vi "Harmonics MSMT Configure Fetch Evaluations.vi"(8 "error in (no error)":errorcluster, 9 "SA Pin":string="SA PIN", 10 "Harmonic":i8, 11 "Harmonics in":refnum<class "Harmonics.lvclass">) -> (0 "error out":errorcluster, 1 "Exported Data Location":string, 2 "Array":T1[](array[typedef]) {"Low Limit" format="%#_13g"; "SI Scaling" items=["femto"=-15, "pico"=-12, "nano"=-9, "micro"=-6, "milli"=-3, "percent"=-2, ""=0, "kilo"=3, "mega"=6, "giga"=9, "tera"=12]}, 3 "Harmonics out":refnum<class "Harmonics.lvclass">)   [LabVIEW 2018, in "Harmonics.lvlib" / "Harmonics.lvclass"]
uses:
  Harmonics.lvclass
  C:/Sequence Automation/Plugins/Measurement Interface.lvlibp/Measurement Interface.lvclass
  Plugins/TestStand API Tools (TSAT).lvlibp/Evaluation Actions/Includes/Controls/TSAT Evaluation.ctl
  Plugins/TestStand API Tools (TSAT).lvlibp/Evaluation Actions/Includes/Controls/TSAT Eval SI Unit Scaling.ctl
  Plugins/TestStand API Tools (TSAT).lvlibp/Evaluation Actions/Includes/Controls/TSAT Evaluation Type.ctl
  Plugins/SeqAuto IEvaluation.lvlibp/SeqAuto IEvaluation.lvclass
  Harmonics.lvclass/Harmonics.ctl
  Evaluations/Harmonics/Harmonics_CHP/Harmonics_CHP.lvclass/Harmonics_CHP.ctl
  Protected Methods/Read DC Pins.vi
  Evaluations/Harmonics/Harmonics_CHP/Read Exported Data Location.vi
  Evaluations/DC Evaluations/DC_IDD.lvclass
  C:/Sequence Automation/Plugins/SeqAuto IEvaluation.lvlibp/SeqAuto IEvaluation.lvclass
  Plugins/Measurement Interface.lvlibp/Private Methods/Measurement Name/Read Measurement Name.vi
  Plugins/Measurement Interface.lvlibp/Private Methods/Measurement Parameters/Read Measurement Parameters.vi
  Plugins/String Database.lvlibp/String Database.lvclass
  Evaluations/Harmonics/Harmonics_CHP/Harmonics_CHP.lvclass
  Plugins/TestStand API Tools (TSAT).lvlibp/Evaluation Actions/TSAT Evaluation Actions.lvlib
  Plugins/Test Number and Bin Generator.lvlibp/Test Number and Bin Generator/Test Number and Bin Generator.lvclass
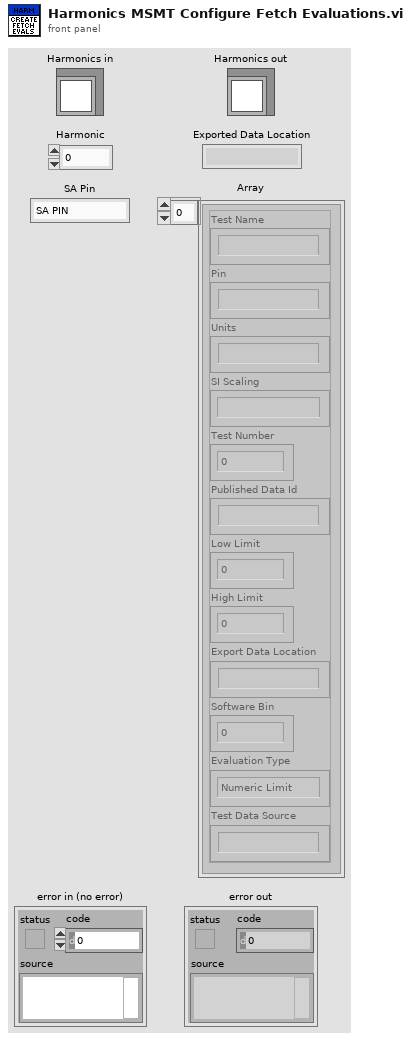
[diagram p1: front panel]
types:
  T1 = typedef "TestStand API Tools (TSAT).lvlibp/TSAT Evaluation Actions.lvlib/TSAT Evaluation.ctl" = cluster{"Test Name":string, "Pin":string, "Units":string, "SI Scaling":T2, "Test Number":i32, "Published Data Id":string, "Low Limit":dbl, "High Limit":dbl, "Export Data Location":string, "Software Bin":i64, "Evaluation Type":T3, "Test Data Source":string}
  T2 = typedef "TestStand API Tools (TSAT).lvlibp/TSAT Evaluation Actions.lvlib/TSAT Eval SI Unit Scaling.ctl" = i16
  T3 = typedef "TestStand API Tools (TSAT).lvlibp/TSAT Evaluation Actions.lvlib/TSAT Evaluation Type.ctl" = enum16{"Numeric Limit", "Pass/Fail", "None"}
  T4 = typedef "Test Number and Bin Generator.lvlibp/Test Number and Bin Generator.lvclass/Session Handle.ctl" = refnum<data-value>
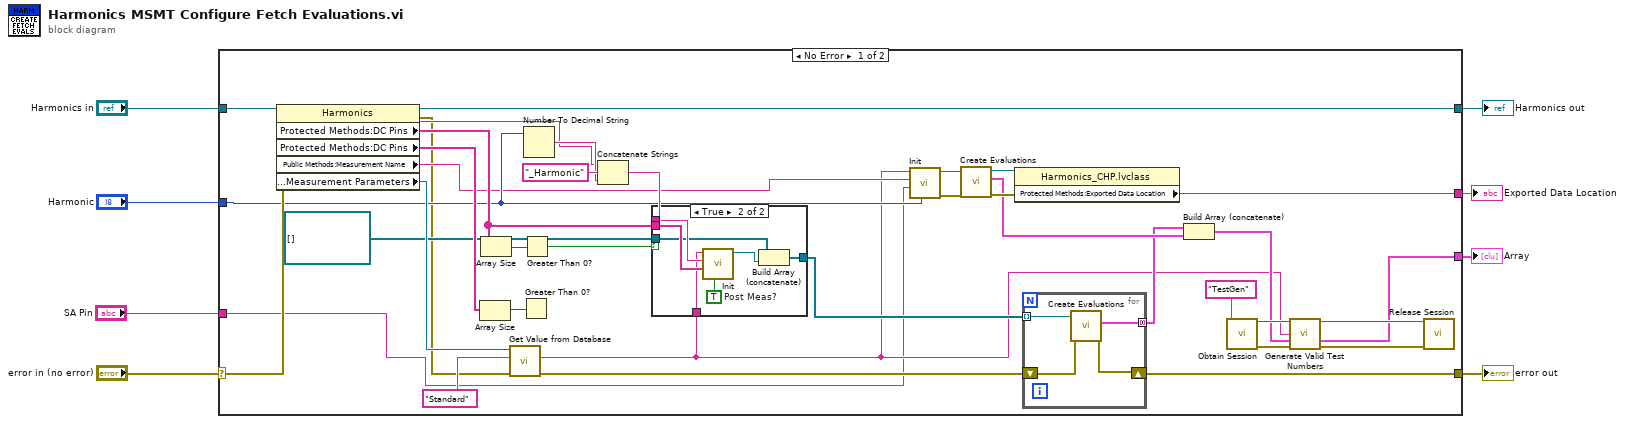
[diagram p0: block diagram]
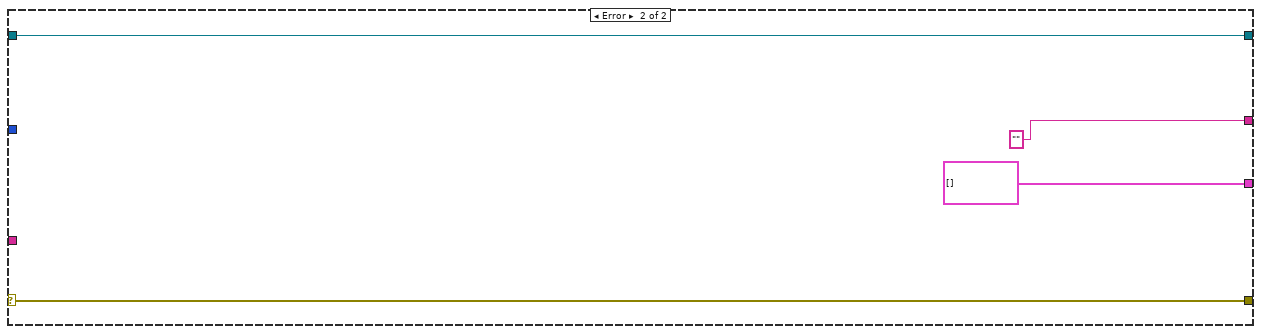
[diagram p3: hidden frame]
diagram:
  n1 = case shown="No Error" "error in (no error)" {
    selector: "error in (no error)" -> [w44 w60]
    tunnel: [w29 w60] -> w7
    tunnel: [w12 w59] -> w5
    tunnel: "Harmonics in" -> [w43 w59]
    tunnel: "Harmonic" -> [w15 _]
    tunnel: [w30 "" ("Protected Methods:Exported Data Location 2")] -> w3
    tunnel: [w20 T1[] []] -> w2
    tunnel: "SA Pin" -> [w9 _]
    frame No Error {
      n2 = property class="Harmonics"(reference=w43, error in=w44) -> (reference out=w12:refnum<class "Harmonics.lvclass">, error out=w10:errorcluster, "Protected Methods:DC Pins"=w38:string[], "Protected Methods:DC Pins"=w42:string[], "Public Methods:Measurement Name"=w13:string, "Protected Methods:Measurement Parameters"=w37:refnum<class "String Database.lvclass">)
      n3 = Array Size(array=w42) -> (size(s)=w40:i32)
      n4 = Array Size(array=w38) -> (size(s)=w41:i32)
      n5 = call "Get Value from Database.vi"("error in (no error)"=w10, "Entry Name"="Standard", "Message in"=w37) -> ("error out"=w19:errorcluster, "Entry Value"=w11:string)  [unwired: 5 in, 2 out]
      n6 = Greater Than 0?(x=w40) -> ()  [unwired: 1 out]
      n7 = Greater Than 0?(x=w41) -> (x > 0?=w39:bool)
      n8 = Number To Decimal String(number=w15) -> (decimal integer string=w14:string)  [unwired: 1 in]
      n9 = Concatenate Strings(w13, "_Harmonic" ("string"), w14) -> (w17:string)
      n10 = case shown="True" w39 {
        tunnel: w17 -> [_ w56]
        tunnel: w38 -> [_ w55]
        tunnel: refnum<class "SeqAuto IEvaluation.lvclass">[] [] -> [w49 w53]
        tunnel: [w49 w52] -> w35
        tunnel: w11 -> [_ w51]
        frame False {
        }
        frame True {
          w50 = TRUE  # Post Meas?
          n11 = call "Init.vi"("Post Meas?"=w50, "DC Pins"=w55, "Measurement Name"=w56, "Standard"=w51) -> ("DC_IDD out"=w54:refnum<class "DC_IDD.lvclass">)  [unwired: 6 in, 1 out]
          n12 = Build Array (concatenate)(w53, w54) -> (w52:refnum<class "SeqAuto IEvaluation.lvclass">[])
        }
      }
      n13 = call "Init.vi"("Harmonic"=w15, "SA Pin"=w9, "Measurement Name"=w13, "Standard"=w11) -> ("error out"=w33:errorcluster, "Harmonics_CHP out"=w34:refnum<class "Harmonics_CHP.lvclass">)  [unwired: 6 in]
      n14 = call-dynamic "Create Evaluations.vi"("error in (no error)"=w33, "IEvaluation in"=w34) -> ("error out"=w31:errorcluster, "Evaluations Out"=w28:T1[], "IEvaluation out"=w32:refnum<class "Harmonics_CHP.lvclass">)  [unwired: 7 in]
      n15 = property class="Harmonics_CHP.lvclass"(reference=w32, error in=w31) -> ("Protected Methods:Exported Data Location"=w30:string)  [unwired: 2 out]
      n16 = for {
        tunnel: w35 -> [w48] mode=indexing
        shift-right: [w46] -> w29
        shift-left: w19 -> [w47]
        tunnel: [w45] -> w27 mode=concatenating
        n17 = call-dynamic "Create Evaluations.vi"("error in (no error)"=w47, "IEvaluation in"=w48) -> ("error out"=w46:errorcluster, "Evaluations Out"=w45:T1[])  [unwired: 7 in, 1 out]
      }
      n18 = Build Array (concatenate)(w27, w28) -> (w21:T1[])
      n19 = call "Obtain Session.vi"("Session  Name ()"="TestGen") -> ("Session Handle"=w25:T4, "error out"=w22:errorcluster)  [unwired: 13 in]
      n20 = call "Generate Valid Test Numbers.vi"("Session Handle in"=w25, "Test Group"=w11, "Evaluations In"=w21, "error in (no error)"=w22) -> ("Session Handle out"=w24:T4, "Evaluations Out"=w20:T1[], "error out"=w23:errorcluster)  [unwired: 9 in]
      n21 = call "Release Session.vi"("Session Handle"=w24, "error in (no error)"=w23) -> ()  [unwired: 13 in, 1 out]
    }
    frame Error {
    }
  }
  "error out" <- w7
  "Harmonics out" <- w5
  "Exported Data Location" <- w3
  "Array" <- w2
